vi "MCList-Clicked cell position.vi"(9 "Coords":T2, 11 "MulticolumnListbox in":refnum<vi>) -> (1 "Cell Position":T1, 3 "MulticolumnListbox out":refnum<vi>)   [LabVIEW 2017]
uses:
  <vilib>/Utility/miscctls.llb/LVPoint32TypeDef.ctl
  <vilib>/Utility/miscctls.llb/LVRowAndColumnTypeDef.ctl
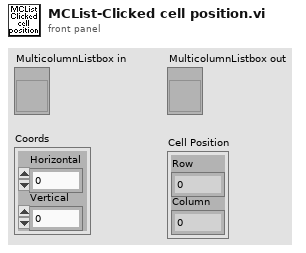
[diagram p1: front panel]
types:
  T1 = typedef "LVRowAndColumnTypeDef.ctl" = cluster{"Row":i32, "Column":i32}
  T2 = typedef "LVPoint32TypeDef.ctl" = cluster{"Horizontal":i32, "Vertical":i32}
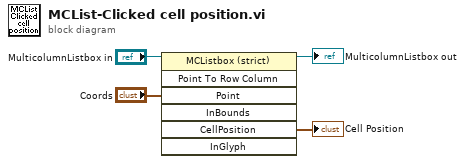
[diagram p0: block diagram]
diagram:
  n1 = invoke on="Invoke Node" class="MCListbox (strict)" method="Point To Row Column"(reference="MulticolumnListbox in", "Point"="Coords") -> (reference out=→"MulticolumnListbox out":refnum<vi>, "CellPosition"=→"Cell Position":T1)  [unwired: 5 in, 5 out]
